vi "Sagar C V Half Subtractor and Full Subtractor.vi"() -> ()   [LabVIEW 2018]
panel:
  in  "?":string
  in  "?":string
  out "Borrow_FS":bool
  out "Difference_FS":bool
  out "Borrow_HS":bool
  out "Difference_HS":bool
  in  "Bin":bool
  in  "B":bool
  in  "A":bool
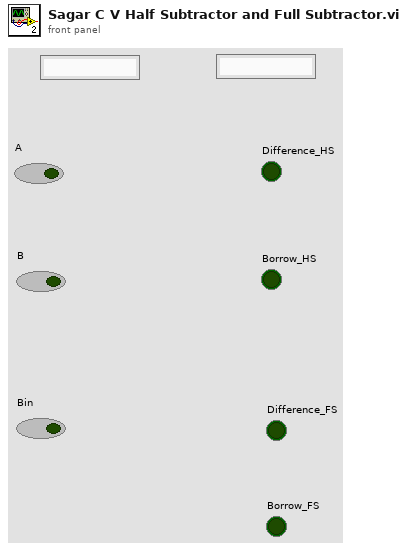
[diagram p1: front panel]
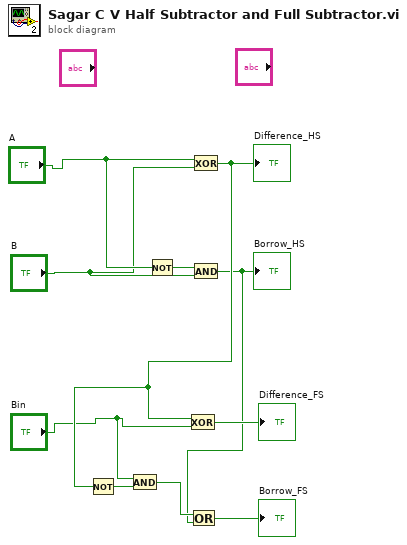
[diagram p0: block diagram]
diagram:
  n1 = Not(x="A") -> (.not. x?=w10:bool)
  n2 = Exclusive Or(1:"B", 2:"A") -> (0:w4:bool)
  "Difference_HS" <- w4
  n3 = Not(x=w4) -> (.not. x?=w5:bool)
  n4 = And(x="Bin", y=w5) -> (x .and. y?=w2:bool)
  n5 = Exclusive Or(1:"Bin", 2:w4) -> (0:→"Difference_FS":bool)
  n6 = And(x=w10, y="B") -> (x .and. y?=w1:bool)
  "Borrow_HS" <- w1
  n7 = Or(x=w2, y=w1) -> (x .or. y?=→"Borrow_FS":bool)
